vi "xcopyYesterday.vi"   [LabVIEW 2012]
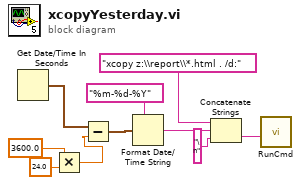
[diagram p0: block diagram]
diagram:
  n1 = Get Date/Time In Seconds() -> (seconds since 1Jan1904=w10:timestamp)
  n2 = Multiply(x=3600.0, y=24.0) -> (x*y=w8:dbl)
  n3 = Subtract(x=w10, y=w8) -> (x-y=w7:timestamp)
  n4 = Format Date/Time String(time format string (%c)="%m-%d-%Y", seconds (now)=w7) -> (date/time string=w4:string)  [unwired: 1 in]
  n5 = Concatenate Strings("xcopy z:\\report\\*.html . /d:" ("string"), w4, "\n" ("string")) -> (w1:string)
  n6 = call "RunCmd.vi"("Cmd String"=w1) -> ()  [unwired: 9 in, 2 out]
